vi "Go To Connected.vi"(7 "error in (no error)":errorcluster, 10 "Receiver.lvlib:Receiver Commands.lvlib:Connect Command.lvlib:Connect Command.lvclass 2":refnum<class "Connect Command.lvclass">) -> (0 "error out":errorcluster, 3 "Receiver State out":refnum<class "State Actor.lvclass">)   [LabVIEW 2013, in "Receiver.lvlib" / "Receive Commands Using State Actors.lvlib" / "Connect Command.lvlib" / "Connect Command.lvclass"]
uses:
  Connect Command.lvclass
  <vilib>/ni/Actors/State Actor/State Actor/State Actor.lvclass
  States/Connected/Connected.lvclass
  <vilib>/ActorFramework/Actor/Actor.lvclass/Actor.ctl
  <vilib>/ActorFramework/Message Enqueuer/Message Enqueuer.lvclass/Message Enqueuer.ctl
  <vilib>/ActorFramework/Message Enqueuer/Enqueue.vi
  <vilib>/ActorFramework/Message Priority Queue/Priority Enqueue.vi
  Command Messages/Complete Command Msg/Complete Command Msg.lvclass
  <vilib>/ActorFramework/Actor/Actor.lvclass
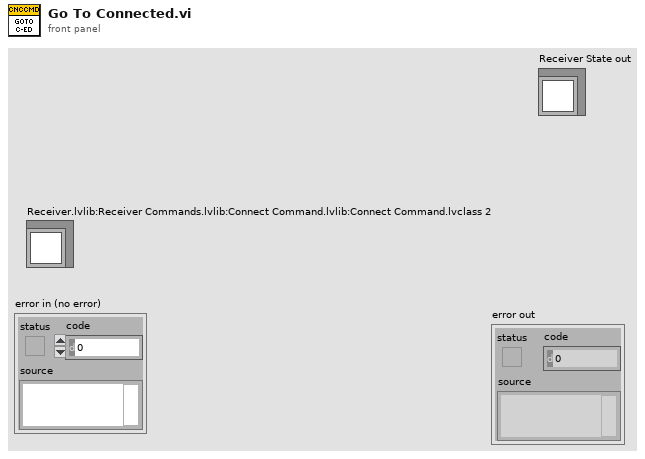
[diagram p1: front panel]
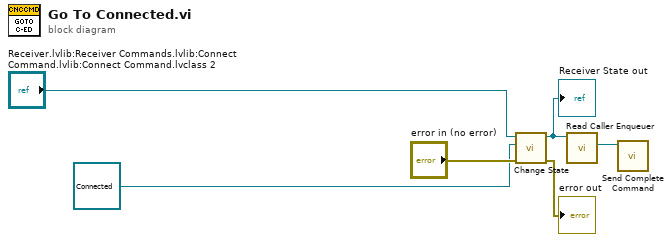
[diagram p0: block diagram]
diagram:
  n1 = call <vilib>:"Change State.vi"("error in (no error)"="error in (no error)", "New State in"=refnum<class "Connected.lvclass"> refnum ("Receiver.lvlib:Receiver Commands.lvlib:Connect Command.lvlib:Executing States.lvlib:Connected.lvclass"), "State in"="Receiver.lvlib:Receiver Commands.lvlib:Connect Command.lvlib:Connect Command.lvclass 2") -> ("error out"=→"error out":errorcluster, "State out"=w4:refnum<class "State Actor.lvclass">)  [unwired: 7 in]
  "Receiver State out" <- w4
  n2 = call <vilib>:"Read Caller Enqueuer.vi"("Actor"=w4) -> ("Caller Enqueuer"=w3:refnum<class "Message Enqueuer.lvclass">)  [unwired: 10 in]
  n3 = call "Send Complete Command.vi"("Message Enqueuer"=w3) -> ()  [unwired: 9 in, 2 out]
